vi "GUI Init.vi"(7 "Ring":refnum<vi>, 8 "error in (no error)":errorcluster, 9 "MuliLB":refnum<vi>, 10 "ListBox":refnum<vi>, 11 "FP Ref":refnum<vi>) -> (0 "error out":errorcluster)   [LabVIEW 2011]
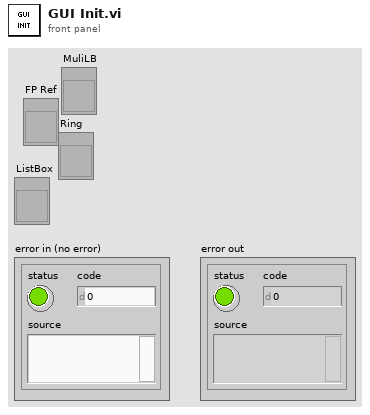
[diagram p1: front panel]
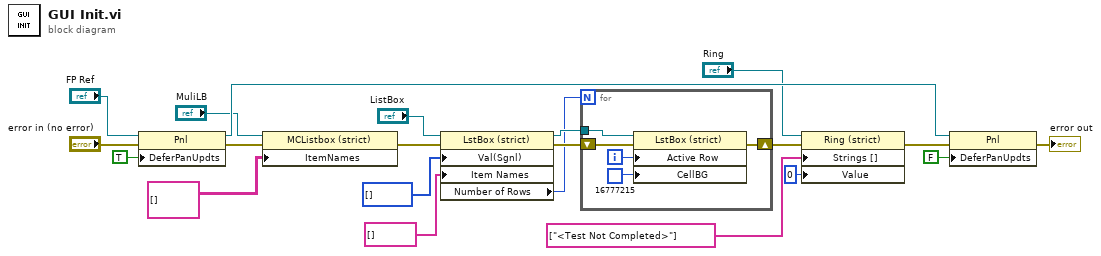
[diagram p0: block diagram]
diagram:
  n1 = property class="Pnl"(reference="FP Ref", error in="error in (no error)", "DeferPanUpdts"=TRUE ("Defer Panel Updates")) -> (reference out=w11:refnum<vi>, error out=w9:errorcluster)
  n2 = property class="MCListbox (strict)"(reference="MuliLB", error in=w9, "ItemNames"=string[][] [] ("Item Names")) -> (error out=w7:errorcluster)  [unwired: 1 out]
  n3 = property on="Property Node" class="LstBox (strict)"(reference="ListBox", error in=w7, "Val(Sgnl)"=i32[] [] ("Value (Signaling)"), "Item Names"=string[] [] ("Value (Signaling)")) -> (reference out=w20:refnum<vi>, error out=w19:errorcluster, "Number of Rows"=w6:u32)
  n4 = for {
    N: w6 -> [_]
    shift-right: [w25] -> w5
    shift-left: w19 -> [w26]
    tunnel: w20 -> [w22]
    i -> [w24]
    n5 = property on="Property Node" class="LstBox (strict)"(reference=w22, error in=w26, "Active Row"=w24, "CellBG"=u32 16777215) -> (error out=w25:errorcluster)  [unwired: 1 out]
  }
  n6 = property on="Property Node" class="Ring (strict)"(reference="Ring", error in=w5, "Strings []"=string[] ["<Test Not Completed>"], "Value"=u16 0) -> (error out=w3:errorcluster)  [unwired: 1 out]
  n7 = property class="Pnl"(reference=w11, error in=w3, "DeferPanUpdts"=FALSE ("Defer Panel Updates")) -> (error out=→"error out":errorcluster)  [unwired: 1 out]
